vi "IMAQdx HL-Sequence.vi"(8 "ErrIn":errorcluster, 9 "Number of images":i32=10, 10 "ImgName":string="untitled", 11 "Camera":refnum<k21> caption="IMAQdx Session") -> (0 "ErrOut":errorcluster, 3 "ImgOut":T1[](array[typedef]))   [LabVIEW 2013]
doc: "Use this template to build a VI to use as a subVI."
uses:
  <vilib>/vision/Image Controls.llb/IMAQ Image.ctl
  <vilib>/vision/driver/NI_Vision_Acquisition_Software.lvlib
panel:
  # "Input Parameters"
  # "Output Parameters"
  # "VI Description:\nThis VI is created to snap a image from imaging device."
  # ":: MVI Framework V1.0 ::\nAuthor:Gaoke Yang\nEmail: gaoke.yang@yahoo.com\nWeb: www.mvicontrol.com\nCopyright (C) 2013, MVI Technologies All Rights Reserved"
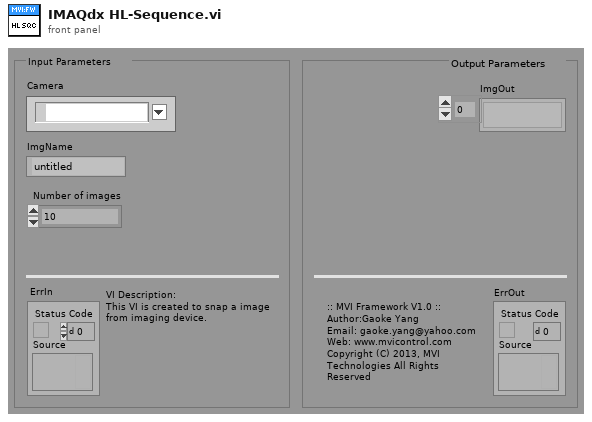
[diagram p1: front panel]
types:
  T1 = typedef "IMAQ Image.ctl" = refnum<image>
  T2 = typedef "IMAQdx.ctl" = refnum<k21>
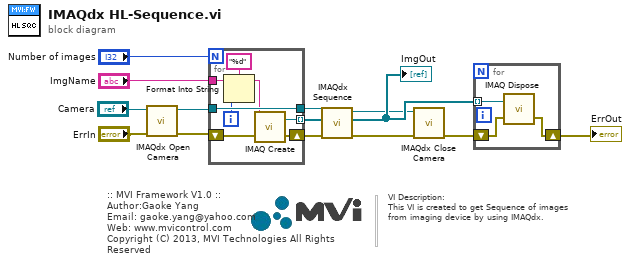
[diagram p0: block diagram]
diagram:
  # "VI Description:\nThis VI is created to get Sequence of images \nfrom imaging device by using IMAQdx."
  # ":: MVI Framework V1.0 ::\nAuthor:Gaoke Yang\nEmail: gaoke.yang@yahoo.com\nWeb: www.mvicontrol.com\nCopyright (C) 2013, MVI Technologies All Rights Reserved"
  n1 = call <vilib>:"IMAQdx Open Camera.vi"("error in"="ErrIn", "Session In"="Camera") -> ("error out"=w3:errorcluster, "Session Out"=w2:T2)  [unwired: 8 in]
  n2 = for {
    N: "Number of images" -> [_]
    tunnel: [w21] -> w8 mode=indexing
    tunnel: w2 -> [w19]
    tunnel: [w19] -> w9
    shift-right: [w22] -> w7
    shift-left: w3 -> [w20]
    tunnel: "ImgName" -> [w15]
    i -> [w18]
    n3 = Format Into String(format string="%d", initial string=w15, w18) -> (resulting string=w17:string)  [unwired: 1 in, 1 out]
    n4 = call "IMAQ Create"("Image Name"=w17, "error in (no error)"=w20) -> ("New Image"=w21:T1, "error out"=w22:errorcluster)  [unwired: 2 in, 1 out]
  }
  n5 = call <vilib>:"IMAQdx Sequence.vi"("error in"=w7, "Images In"=w8, "Session In"=w9) -> ("error out"=w5:errorcluster, "Images Out"=w4:T1[], "Session Out"=w1:T2)  [unwired: 6 in]
  "ImgOut" <- w4
  n6 = call <vilib>:"IMAQdx Close Camera.vi"("error in"=w5, "Session In"=w1) -> ("error out"=w6:errorcluster)  [unwired: 9 in]
  n7 = for {
    tunnel: w4 -> [w25] mode=indexing
    shift-right: [w23] -> w12
    shift-left: w6 -> [w24]
    n8 = call "IMAQ Dispose"("Image"=w25, "error in (no error)"=w24) -> ("error out"=w23:errorcluster)  [unwired: 1 in, 3 out]
  }
  "ErrOut" <- w12
